vi "TA_Plot_Spectra_1.vi"(10 "DeltaA (mOD)":dbl[][](array[numeric])=array214x154[32956 elements], 11 "Wavelength (nm)":dbl[](array[numeric])=[410.231567, 411.880432, 413.529175, 415.177826, 416.826385, 418.474854, 420.123199, 421.771484, 423.419617, 425.067688, 426.715637, 428.363495, 430.01123, 431.658905, 433.306458, 434.953888, 436.601227, 438.248474, 439.89563, 441.542633, 443.189575, 444.836365, 446.483124, 448.1297, 449.776215, 451.422607, 453.068909, 454.715118, 456.361176, 458.007111, 459.653015, 461.298798, 462.944397, 464.589966, 466.235382, 467.880707, 469.52594, 471.171021, 472.815979, 474.460876, 476.105682, 477.750305, 479.394836, 481.039276, 482.683624, 484.327789, 485.971893, 487.615875, 489.259766, 490.903503, 492.54715, 494.190674, 495.834076, 497.477386, 499.120544, 500.763611, 502.406555, 504.049408, 505.692108, 507.334686, 508.977173, 510.619537, 512.261719, 513.90387, 515.545898, 517.187805, 518.82959, 520.471191, 522.112732, 523.754089, 525.395447, 527.036499, 528.677612, 530.318481, 531.959351, 533.599976, 535.24054, 536.88092, 538.521301, 540.161438, 541.801453, 543.441406, 545.081238, 546.720886, 548.360535, 549.999878, 551.639221, 553.278442, 554.917358, 556.556274, 558.195129, 559.833862, 561.472412, 563.110779, 564.749023, 566.387207, 568.025208, 569.663025, 571.300842, 572.938477, 574.575989, 576.213379, 577.850586, 579.487732, 581.124634, 582.761414, 584.398193, 586.03479, 587.671265, 589.307495, 590.943726, 592.579712, 594.215637, 595.851318, 597.487, 599.122498, 600.757874, 602.393066, 604.028259, 605.663208, 607.297913, 608.932617, 610.567078, 612.201538, 613.835815, 615.46991, 617.103943, 618.737793, 620.37146, 622.004944, 623.638428, 625.271667, 626.904846, 628.537781, 630.170715, 631.803406, 633.435974, 635.06842, 636.700623, 638.332764, 639.964783, 641.596619, 643.228333, 644.859924, 646.491272, 648.12262, 649.753662, 651.384644, 653.015442, 654.646179, 656.276672, 657.907104, 659.537292, 661.167419, 662.797302, 664.427124, 666.056702, 667.686218, 669.315552, 670.944763, 672.573792, 674.202759, 675.831421, 677.460022, 679.08844, 680.716736, 682.344849, 683.972839, 685.600708, 687.228333, 688.855896, 690.483215, 692.110413, 693.737488, 695.364319, 696.991028, 698.617676, 700.24408, 701.870361, 703.49646, 705.122375, 706.74823, 708.373779, 709.999268, 711.624634, 713.249817, 714.874817, 716.499634, 718.124329, 719.74884, 721.37323, 722.997375, 724.62146, 726.2453, 727.86908, 729.492615, 731.116028, 732.739197, 734.362244, 735.985168, 737.60791, 739.230469, 740.852905, 742.475098, 744.097229, 745.719177, 747.34082, 748.962402, 750.583801, 752.205078, 753.826172, 755.447083, 757.06781, 758.688416]) -> (3 "TA Spectra":cluster{"Array":dbl[], "Array 2":dbl[]}[](graph))   [LabVIEW 2025]
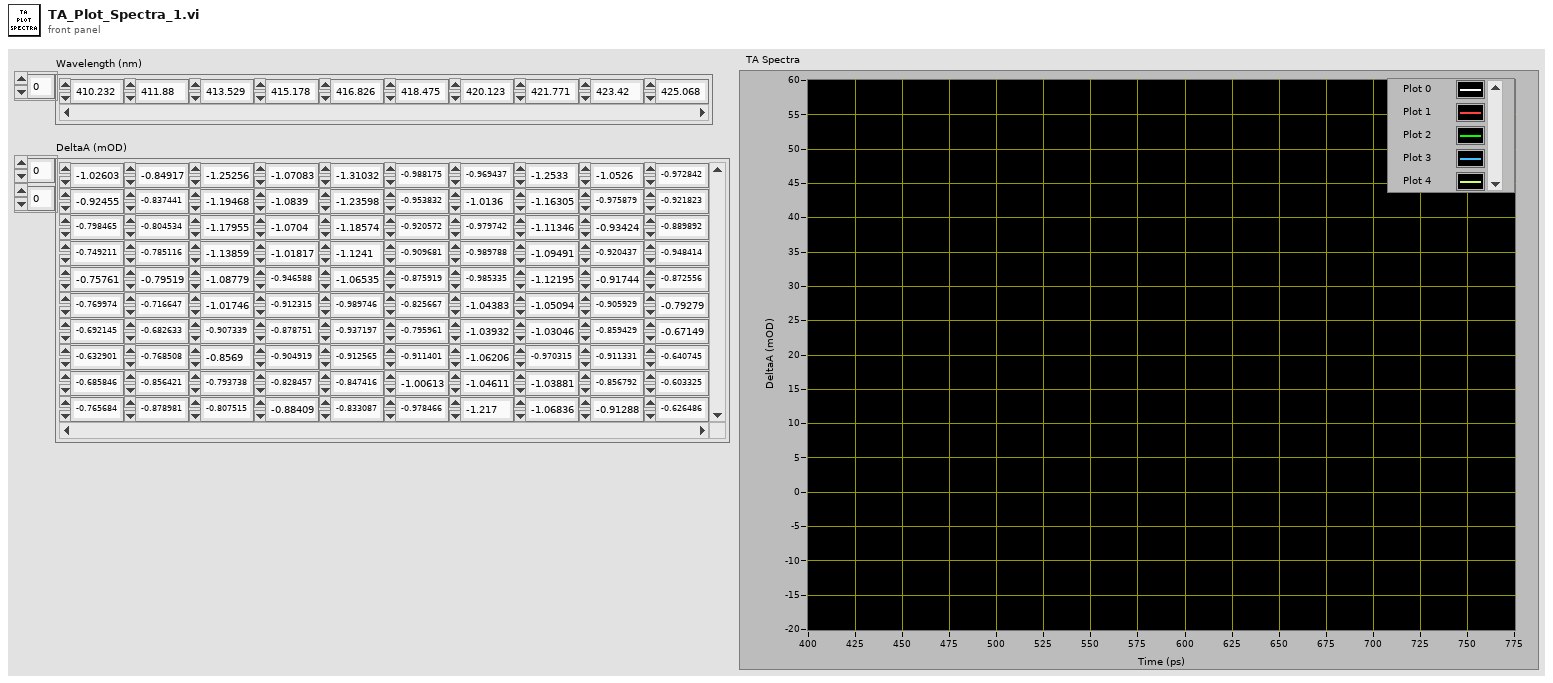
[diagram p1: front panel]
types:
  T1 = cluster{"Wavelength (nm)":dbl[], "DeltaA (mOD)":dbl[]}
  T2 = cluster{"Wavelength (nm)":dbl[], "DeltaA (mOD)":dbl[]}[]
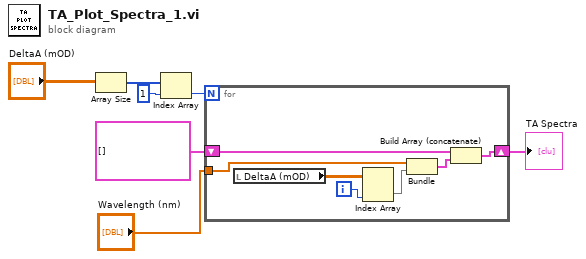
[diagram p0: block diagram]
diagram:
  n1 = Array Size(array="DeltaA (mOD)") -> (size(s)=w4:i32[])
  n2 = Index Array(array=w4, index=1) -> (element=w5:i32)
  n3 = for {
    N: w5 -> [_]
    tunnel: "Wavelength (nm)" -> [w14]
    shift-right: [w10] -> w1
    shift-left: cluster{"Array":dbl[], "Array 2":dbl[]}[] [] ("Array") -> [w9]
    i -> [w8]
    n4 = local read "DeltaA (mOD)"() -> (w12:dbl[][])
    n5 = Index Array(array=w12, index (col)=w8) -> (element=w13:dbl[])  [unwired: 1 in]
    n6 = Bundle("Wavelength (nm)"=w14, "DeltaA (mOD)"=w13) -> (w11:T1)  [unwired: 1 in]
    n7 = Build Array (concatenate)(w9, w11) -> (w10:T2)
  }
  "TA Spectra" <- w1
